vi "Magnetic Sweep 1.1.vi"() -> ()   [LabVIEW 2011]
panel:
  out "Intensity Graph 2":dbl[][](graph)
  in  "stop":bool
  out "error out 3":errorcluster
  out "error out 2":errorcluster
  out "Intensity Graph":dbl[][](graph)
  in  "Contour plot (ramp down)":path
  in  "Raw data (ramp down)":path
  out "Elapsed Time (s)":dbl
  out "Numeric":i32
  in  "error out":errorcluster
  out "Initial Temperature":string
  out "Zero field reached":bool
  out "Target field reached":bool
  in  "Upper limite":dbl
  in  "Temperature\nramping step":dbl
  in  "Heater range":i16(ring) items=["High", "Medium", "Low"]
  in  "D gain":dbl
  in  "I gain":dbl
  in  "P gain":dbl
  in  "Contour plot (ramp up)":path
  out "Time elapsed":string
  in  "Timer":bool caption="Reset"
  in  "date format":enum16{"short", "long", "abbreviated"}(ring)
  in  "Save":bool
  in  "Raw data (ramp  up)":path
  out "Temperature vs Time":cluster{dbl[], dbl[]}(graph)
  out "current time":timestamp
  out "Magnetic\nField":cluster{dbl[], dbl[]}(graph)
  out "Current Resistance":string
  out "Current Temperature":string
  out "Current Field":string
  out "Status":string
  in  "Field Sweep":bool
  in  "Start":bool
  out "Parameter\nSetup":string
  in  "Ramp rate":dbl
  in  "Traget Field":dbl
  out "Init Response":string
  in  "error in (no error)":errorcluster
  in  "IP Address":string
  in  "Ramp":bool
  in  "Update":bool
  in  "Ramp to Zero":bool
  in  "P Switch":bool
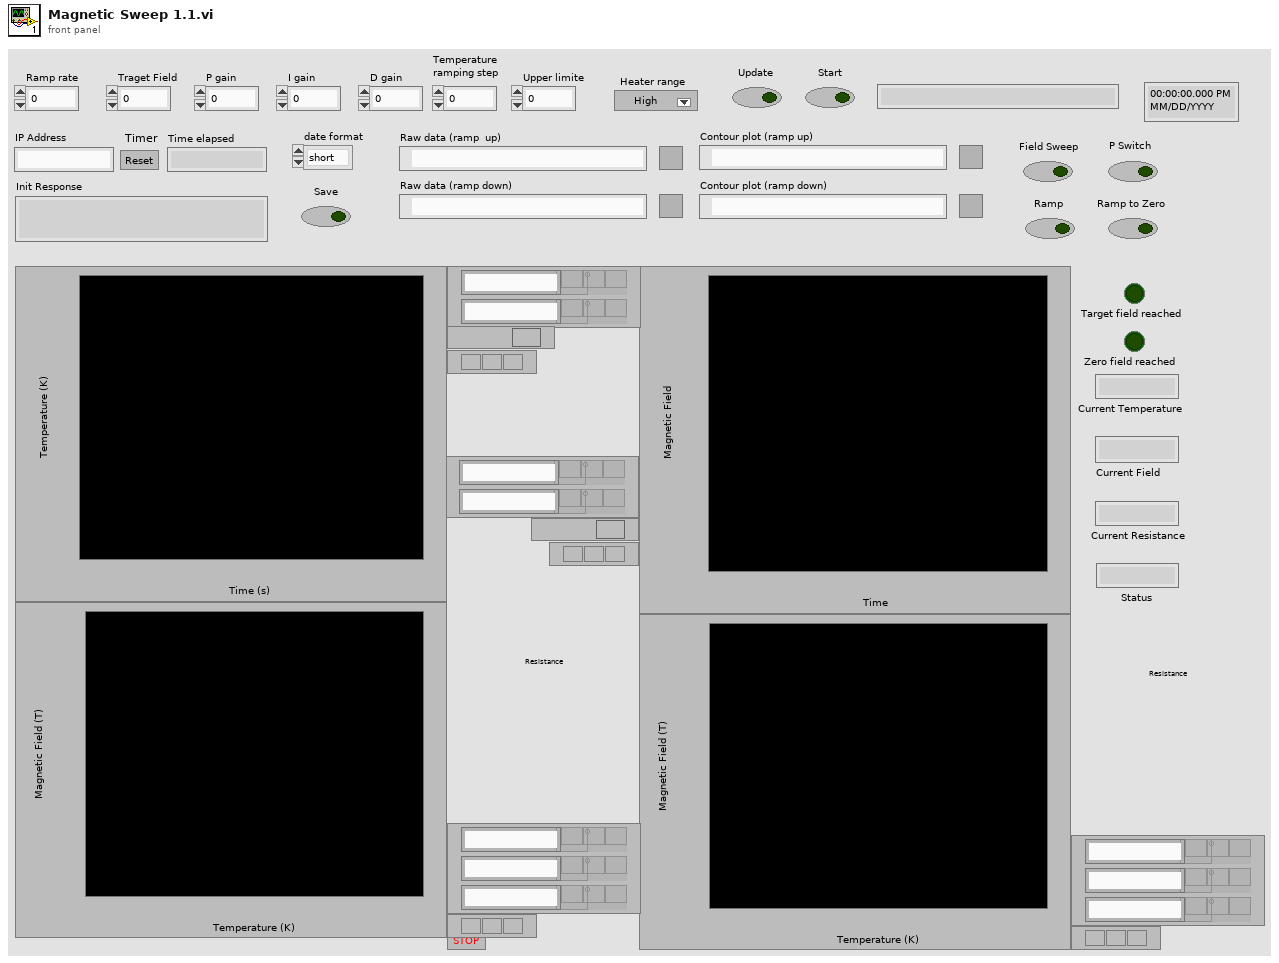
[diagram p1: front panel]
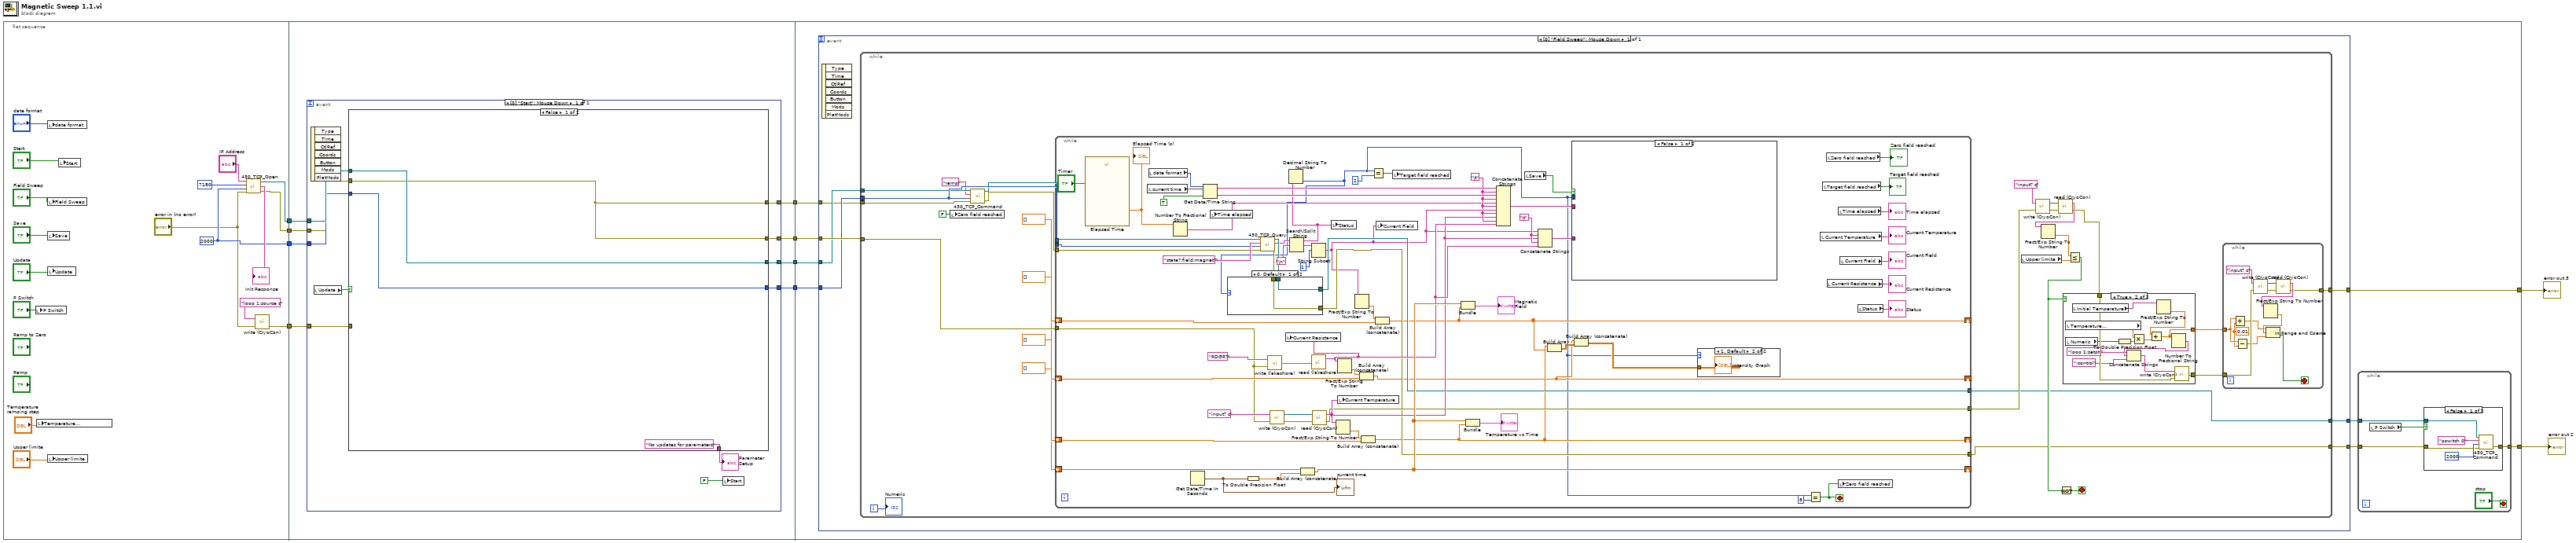
[diagram p0: block diagram]
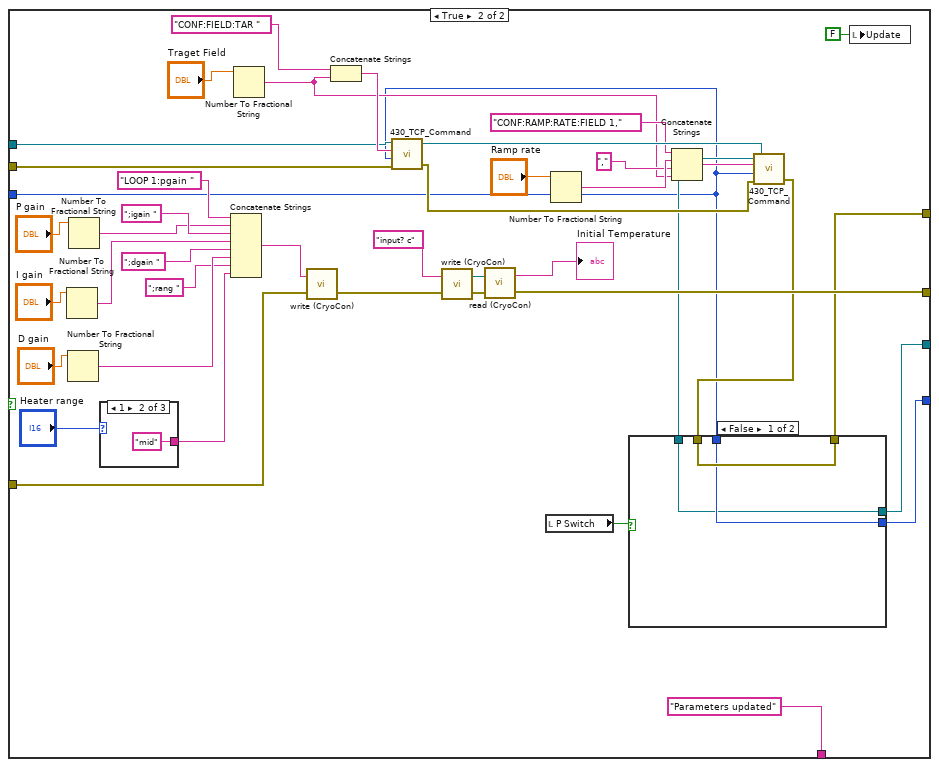
[diagram p2: hidden frame]
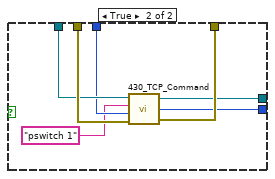
[diagram p3: hidden frame]
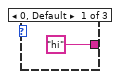
[diagram p4: hidden frame]
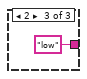
[diagram p5: hidden frame]
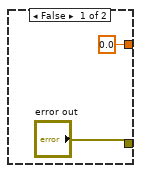
[diagram p7: hidden frame]
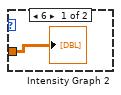
[diagram p8: hidden frame]
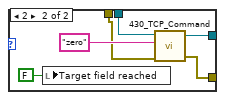
[diagram p9: hidden frame]
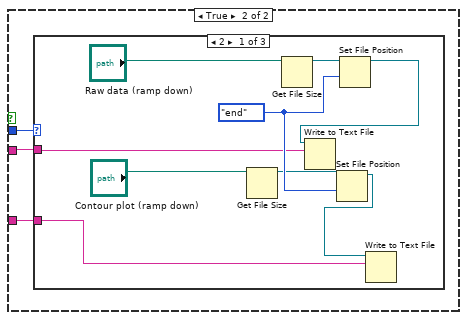
[diagram p10: hidden frame]
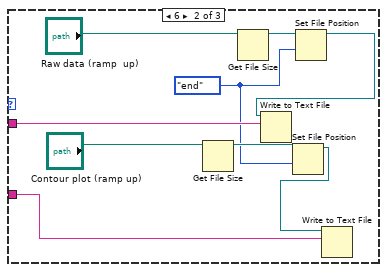
[diagram p11: hidden frame]
diagram:
  n1 = flat-sequence {
    tunnel: [w23] -> w10
    tunnel: [w22] -> w9
    tunnel: [w21] -> w8
    tunnel: [w17] -> w5
    tunnel: w10 -> [w35]
    tunnel: w9 -> [w34]
    tunnel: w8 -> [w33]
    tunnel: [w32] -> w7
    tunnel: [w31] -> w6
    tunnel: w5 -> [w30]
    tunnel: [w29] -> w4
    tunnel: [w28] -> w3
    tunnel: w7 -> [w113]
    tunnel: w6 -> [w112]
    tunnel: w4 -> [w111]
    tunnel: w3 -> [w110]
    tunnel: [w109] -> w2
    tunnel: [w107] -> w1
    frame #0 {
      w22 = 2000 ("Timeout")
      n2 = local write "P Switch"("P Switch") -> ()
      n3 = local write "Temperature\nramping step"("Temperature\nramping step") -> ()
      n4 = local write "date format"("date format") -> ()
      n5 = local write "Field Sweep"("Field Sweep") -> ()
      n6 = local write "Save"("Save") -> ()
      n7 = local write "Update"("Update") -> ()
      n8 = local write "Upper limite"("Upper limite") -> ()
      n9 = local write "Start"("Start") -> ()
      n10 = call "430_TCP_Open.vi"("IP Address"="IP Address", "TCP Port"=7180, "timeout ms (2000)"=w22, "error in (no error)"="error in (no error)") -> ("connection ID"=w23:refnum<k5>, "Init Response"=→"Init Response":string, "error out"=w21:errorcluster)  [unwired: 2 in]
      n11 = call "write (CryoCon).vi"("error in (no error)"="error in (no error)", "write buffer"="loop 1:source c") -> ("error out"=w17:errorcluster)  [unwired: 1 out]
    }
    frame #1 {
      n12 = event shown="[0] \"Start\": Mouse Down" {
        selector: _ -> [_]
        dyn-events: _ -> [_]
        timeout: _ -> [_]
        tunnel: w35 -> [w45]
        tunnel: w34 -> [w44]
        tunnel: w33 -> [w43]
        tunnel: [w42] -> w32
        tunnel: [w41] -> w31
        tunnel: w30 -> [w38]
        tunnel: [w37] -> w29
        tunnel: [w36] -> w28
        event "Start": Mouse Down {
          n13 = event-data() -> ()  [unwired: 1 in, 7 out]
          n14 = local read "Update"() -> (w46:bool)
          n15 = case shown="False" w46 {
            tunnel: w45 -> [w50 w90]
            tunnel: w44 -> [w49 w53]
            tunnel: w43 -> [w47 w78]
            tunnel: [w50 w52] -> w42
            tunnel: [w49 w51] -> w41
            tunnel: ["No updates for parameters" ("String") "Parameters updated" ("String")] -> w39
            tunnel: w38 -> [_ w67]
            tunnel: [w47 w59] -> w37
            tunnel: [w47 w55] -> w36
            frame False {
            }
            frame True {
              n16 = Number To Fractional String(number="I gain") -> (F-format string=w71:string)  [unwired: 3 in]
              n17 = Number To Fractional String(number="D gain") -> (F-format string=w69:string)  [unwired: 3 in]
              n18 = Number To Fractional String(number="P gain") -> (F-format string=w72:string)  [unwired: 3 in]
              n19 = case shown="1" "Heater range" {
                tunnel: ["hi" "mid" "low"] -> w64
                frame 0, Default {
                }
                frame 1 {
                }
                frame 2 {
                }
              }
              n20 = Concatenate Strings("LOOP 1:pgain " ("write buffer"), w72, ";igain " ("string"), w71, ";dgain " ("string"), w69, ";rang " ("string"), w64) -> (w68:string)
              n21 = Number To Fractional String(number="Traget Field") -> (F-format string=w79:string)  [unwired: 3 in]
              n22 = call "write (CryoCon).vi"("error in (no error)"=w67, "write buffer"=w68) -> ("error out"=w60:errorcluster)  [unwired: 1 out]
              n23 = Concatenate Strings("CONF:FIELD:TAR ", w79) -> (w91:string)
              n24 = call "430_TCP_Command.vi"("error in (no error)"=w78, "Timeout"=w53, "Command"=w91, "connection ID"=w90) -> ("error out"=w89:errorcluster, "connection ID out"=w85:refnum<k5>)  [unwired: 1 out]
              n25 = call "write (CryoCon).vi"("error in (no error)"=w60, "write buffer"="input? c") -> ("error out"=w63:errorcluster, "VISA resource name out"=w62:refnum<visa-resource-name>)
              n26 = call "read (CryoCon).vi"("error in (no error)"=w63, "VISA resource name"=w62) -> ("error out"=w59:errorcluster, "read buffer"=→"Initial Temperature":string)
              n27 = local read "P Switch"() -> (w57:bool)
              n28 = Number To Fractional String(number="Ramp rate") -> (F-format string=w83:string)  [unwired: 3 in]
              n29 = Concatenate Strings("CONF:RAMP:RATE:FIELD 1," ("string"), w83, "," ("string"), w79) -> (w86:string)
              n30 = call "430_TCP_Command.vi"("error in (no error)"=w89, "Timeout"=w53, "Command"=w86, "connection ID"=w85) -> ("error out"=w56:errorcluster, "connection ID out"=w54:refnum<k5>)  [unwired: 1 out]
              n31 = case shown="False" w57 {
                tunnel: w56 -> [w95 w102]
                tunnel: [w95 w101] -> w55
                tunnel: w54 -> [w93 w100]
                tunnel: w53 -> [w94 w99]
                tunnel: [w93 w98] -> w52
                tunnel: [w94 w97] -> w51
                frame False {
                }
                frame True {
                  n32 = call "430_TCP_Command.vi"("error in (no error)"=w102, "Timeout"=w99, "Command"="pswitch 1", "connection ID"=w100) -> ("error out"=w101:errorcluster, "bytes written"=w97:i32, "connection ID out"=w98:refnum<k5>)
                }
              }
              n33 = local write "Update"(FALSE ("Update")) -> ()
            }
          }
          "Parameter\nSetup" <- w39
          n34 = local write "Start"(FALSE ("Set Parameter")) -> ()
        }
      }
    }
    frame #2 {
      n35 = event shown="[0] \"Field Sweep\": Mouse Down" {
        selector: _ -> [_]
        dyn-events: _ -> [_]
        timeout: _ -> [_]
        tunnel: w113 -> [w130]
        tunnel: w112 -> [w129]
        tunnel: w111 -> [w131]
        tunnel: w110 -> [w128]
        tunnel: [w127] -> w109
        tunnel: [w126] -> w108
        tunnel: [w125] -> w106
        event "Field Sweep": Mouse Down {
          n36 = event-data() -> ()  [unwired: 1 in, 7 out]
          n37 = while {
            tunnel: w131 -> [w154]
            tunnel: w129 -> [w158]
            tunnel: w130 -> [w157]
            tunnel: w128 -> [w155]
            tunnel: [w134] -> w127
            tunnel: [w133] -> w126
            tunnel: [w132] -> w125
            i -> [w151]
            stop <- w136 stop-if-true
            n38 = local write "Zero field reached"(FALSE ("Zero field reached")) -> ()
            n39 = call "430_TCP_Command.vi"("error in (no error)"=w155, "Timeout"=w158, "Command"="ramp", "connection ID"=w157) -> ("error out"=w159:errorcluster, "connection ID out"=w156:refnum<k5>)  [unwired: 1 out]
            n40 = while {
              shift-right: [w190] -> _
              shift-left: dbl[] [] -> [w242]
              shift-right: [w191] -> _
              shift-left: dbl[] [] -> [w247]
              shift-right: [w188] -> _
              shift-left: dbl[] [] -> [w244]
              shift-right: [w237] -> _
              shift-left: dbl[] [] -> [w238]
              tunnel: w159 -> [w226]
              tunnel: w158 -> [w202]
              tunnel: w156 -> [w225]
              tunnel: w154 -> [w219]
              tunnel: [w212] -> w137
              tunnel: [w200] -> w133
              tunnel: [w199] -> w132
              stop <- w204 stop-if-true
              w230 = "\t"
              w231 = "\t"
              n41 = call "Elapsed Time"("Reset"="Timer") -> ("Elapsed Time (s)"=w217:dbl)  [unwired: 11 in, 7 out]
              "Elapsed Time (s)" <- w217
              n42 = local read "current time"() -> (w228:timestamp)
              n43 = local read "date format"() -> (w220:enum16{"short", "long", "abbreviated"})
              n44 = Number To Fractional String(number=w217) -> (F-format string=w223:string)  [unwired: 3 in]
              n45 = Get Date/Time In Seconds() -> (seconds since 1Jan1904=w216:timestamp)
              "current time" <- w216
              n46 = Get Date/Time String(date format (0)=w220, seconds (now)=w228, want seconds? (F)=TRUE) -> (date string=w233:string, time string=w232:string)
              n47 = local write "Time elapsed"(w223) -> ()
              n48 = To Double Precision Float(number=w216) -> (double precision float=w239:dbl)
              n49 = call "430_TCP_Query.vi"("error in (no error)"=w226, "Timeout"=w202, "Command"="state?;field:magnet?", "connection ID"=w225) -> ("error out"=w214:errorcluster, "Response"=w198:string, "connection ID out"=w203:refnum<k5>)  [unwired: 3 in, 2 out]
              n50 = call "write (lakeshore).vi"("error in (no error)"=w219, "write buffer"="RDGR?") -> ("error out"=w246:errorcluster)
              n51 = call "write (CryoCon).vi"("error in (no error)"=w219, "write buffer"="input? c") -> ("error out"=w248:errorcluster, "VISA resource name out"=w249:refnum<visa-resource-name>)
              n52 = Search/Split String(string=w198, search string/char (-)="\n") -> (substring before match=w197:string, match + rest of string=w196:string)  [unwired: 1 in, 1 out]
              n53 = Decimal String To Number(string=w197) -> (number=w187:i32)  [unwired: 2 in, 1 out]
              n54 = case shown="0, Default" w187 {
                tunnel: w214 -> [w255 w260]
                tunnel: [w255 w259] -> w199
                tunnel: w203 -> [w254 w257]
                tunnel: [w254 w256] -> w200
                frame 0, Default {
                }
                frame 2 {
                  n55 = local write "Target field reached"(FALSE ("Target field reached")) -> ()
                  n56 = call "430_TCP_Command.vi"("error in (no error)"=w260, "Command"="zero", "connection ID"=w257) -> ("error out"=w259:errorcluster, "connection ID out"=w256:refnum<k5>)  [unwired: 1 in, 1 out]
                }
              }
              n57 = Build Array (concatenate)(w238, w239) -> (w237:dbl[])
              n58 = call "read (lakeshore).vi"("error in (no error)"=w246) -> ("read buffer"=w222:string)  [unwired: 1 out]
              n59 = local write "Current Resistance"(w222) -> ()
              n60 = String Subset(string=w196, offset (0)=1) -> (substring=w194:string)  [unwired: 1 in]
              n61 = call "read (CryoCon).vi"("error in (no error)"=w248, "VISA resource name"=w249) -> ("error out"=w212:errorcluster, "read buffer"=w221:string)
              n62 = local write "Status"(w197) -> ()
              n63 = Fract/Exp String To Number(string=w221) -> (number=w241:dbl)  [unwired: 3 in, 1 out]
              n64 = Fract/Exp String To Number(string=w222) -> (number=w240:dbl)  [unwired: 3 in, 1 out]
              n65 = local write "Current Temperature"(w221) -> ()
              n66 = Fract/Exp String To Number(string=w194) -> (number=w243:dbl)  [unwired: 3 in, 1 out]
              n67 = Build Array (concatenate)(w240, w244) -> (w188:dbl[])
              n68 = Build Array (concatenate)(w241, w247) -> (w191:dbl[])
              n69 = Equal?(x=w187, y=2) -> (x = y?=w224:bool)
              n70 = Build Array (concatenate)(w243, w242) -> (w190:dbl[])
              n71 = local write "Current Field"(w194) -> ()
              n72 = local write "Target field reached"(w224) -> ()
              n73 = Bundle(w237, w190) -> (→"Magnetic\nField":cluster{dbl[], dbl[]})  [unwired: 1 in]
              n74 = Bundle(w237, w191) -> (→"Temperature vs Time":cluster{dbl[], dbl[]})  [unwired: 1 in]
              n75 = Concatenate Strings(w233, w231, w232, w231, w223, w231, w194, w231, w221, w231, w222) -> (w236:string)
              n76 = local read "Save"() -> (w215:bool)
              n77 = Concatenate Strings(w194, w230, w221, w230, w222) -> (w229:string)
              n78 = Build Array(w191, w190) -> (w201:dbl[][])
              n79 = case shown="False" w215 {
                tunnel: w236 -> [_ w264]
                tunnel: w229 -> [_ w263]
                tunnel: w187 -> [_ w262]
                frame False {
                }
                frame True {
                  n80 = case shown="2" w262 {
                    tunnel: w264 -> [w266 w282 _]
                    tunnel: w263 -> [w265 w276 _]
                    frame 2 {
                      w272 = enum16{"start", "end", "current"}."end" ("from (0:start)")
                      n81 = Get File Size(file="Contour plot (ramp down)") -> (refnum out=w271:refnum<file>)  [unwired: 1 in, 2 out]
                      n82 = Get File Size(file="Raw data (ramp down)") -> (refnum out=w268:refnum<file>)  [unwired: 1 in, 2 out]
                      n83 = Set File Position(refnum=w271, from (0:start)=w272) -> (refnum out=w273:refnum<file>)  [unwired: 2 in, 1 out]
                      n84 = Set File Position(refnum=w268, from (0:start)=w272) -> (refnum out=w269:refnum<file>)  [unwired: 2 in, 1 out]
                      n85 = Write to Text File(file (use dialog)=w269, text=w266) -> ()  [unwired: 2 in, 3 out]
                      n86 = Write to Text File(file (use dialog)=w273, text=w265) -> ()  [unwired: 2 in, 3 out]
                    }
                    frame 6 {
                      w275 = enum16{"start", "end", "current"}."end" ("from (0:start)")
                      n87 = Get File Size(file="Contour plot (ramp up)") -> (refnum out=w277:refnum<file>)  [unwired: 1 in, 2 out]
                      n88 = Get File Size(file="Raw data (ramp  up)") -> (refnum out=w280:refnum<file>)  [unwired: 1 in, 2 out]
                      n89 = Set File Position(refnum=w277, from (0:start)=w275) -> (refnum out=w274:refnum<file>)  [unwired: 2 in, 1 out]
                      n90 = Set File Position(refnum=w280, from (0:start)=w275) -> (refnum out=w279:refnum<file>)  [unwired: 2 in, 1 out]
                      n91 = Write to Text File(file (use dialog)=w279, text=w282) -> ()  [unwired: 2 in, 3 out]
                      n92 = Write to Text File(file (use dialog)=w274, text=w276) -> ()  [unwired: 2 in, 3 out]
                    }
                    frame Default {
                    }
                  }
                }
              }
              n93 = Build Array (concatenate)(w188, w201) -> (w189:dbl[][])
              n94 = case shown="1, Default" w187 {
                tunnel: w189 -> [w252 w253]
                frame 6 {
                  "Intensity Graph 2" <- w252
                }
                frame 1, Default {
                  "Intensity Graph" <- w253
                }
              }
              n95 = Equal?(x=w187, y=8) -> (x = y?=w204:bool)
              n96 = local read "Current Temperature"() -> (→"Current Temperature":string)
              n97 = local read "Target field reached"() -> (→"Target field reached":bool)
              n98 = local read "Zero field reached"() -> (→"Zero field reached":bool)
              n99 = local read "Current Resistance"() -> (→"Current Resistance":string)
              n100 = local read "Time elapsed"() -> (→"Time elapsed":string)
              n101 = local write "Zero field reached"(w204) -> ()
              n102 = local read "Current Field"() -> (→"Current Field":string)
              n103 = local read "Status"() -> (→"Status":string)
            }
            n104 = local read "Upper limite"() -> (w139:dbl)
            n105 = call "write (CryoCon).vi"("error in (no error)"=w137, "write buffer"="input? c") -> ("error out"=w142:errorcluster, "VISA resource name out"=w143:refnum<visa-resource-name>)
            n106 = call "read (CryoCon).vi"("error in (no error)"=w142, "VISA resource name"=w143) -> ("error out"=w140:errorcluster, "read buffer"=w141:string)
            n107 = Fract/Exp String To Number(string=w141) -> (number=w138:dbl)  [unwired: 3 in, 1 out]
            n108 = Less Or Equal?(x=w138, y=w139) -> (x <= y?=w135:bool)
            n109 = Not(x=w135) -> (.not. x?=w136:bool)
            n110 = case shown="True" w135 {
              tunnel: w140 -> [_ w183]
              tunnel: ["error out" w180] -> w153
              tunnel: [0.0 w179] -> w152
              frame False {
              }
              frame True {
                n111 = local read "Temperature\nramping step"() -> (w177:dbl)
                n112 = local read "Numeric"() -> (w175:i32)
                n113 = local read "Initial Temperature"() -> (w182:string)
                n114 = To Double Precision Float(number=w175) -> (double precision float=w176:dbl)
                n115 = Multiply(x=w177, y=w176) -> (x*y=w178:dbl)
                n116 = Fract/Exp String To Number(string=w182) -> (number=w181:dbl)  [unwired: 3 in, 1 out]
                n117 = Add(x=w181, y=w178) -> (x+y=w179:dbl)
                n118 = Number To Fractional String(number=w179) -> (F-format string=w184:string)  [unwired: 3 in]
                n119 = Concatenate Strings("loop 1:setpt " ("write buffer"), w184, ";control" ("string")) -> (w186:string)
                n120 = call "write (CryoCon).vi"("error in (no error)"=w183, "write buffer"=w186) -> ("error out"=w180:errorcluster)  [unwired: 1 out]
              }
            }
            n121 = while {
              tunnel: w153 -> [w170]
              tunnel: w152 -> [w165]
              tunnel: [w160] -> w134
              stop <- w161 stop-if-true
              w162 = 0.01 ("y")
              n122 = Add(x=w165, y=w162) -> (x+y=w164:dbl)
              n123 = Subtract(x=w165, y=w162) -> (x-y=w163:dbl)
              n124 = call "write (CryoCon).vi"("error in (no error)"=w170, "write buffer"="input? c") -> ("error out"=w169:errorcluster, "VISA resource name out"=w171:refnum<visa-resource-name>)
              n125 = call "read (CryoCon).vi"("error in (no error)"=w169, "VISA resource name"=w171) -> ("error out"=w160:errorcluster, "read buffer"=w167:string)
              n126 = Fract/Exp String To Number(string=w167) -> (number=w166:dbl)  [unwired: 3 in, 1 out]
              n127 = In Range and Coerce(upper limit=w164, x=w166, lower limit=w163) -> (In Range?=w161:bool)  [unwired: 1 out]
            }
            "Numeric" <- w151
          }
        }
      }
      n128 = while {
        tunnel: w108 -> [w118]
        tunnel: [w116] -> w107
        tunnel: w106 -> [w115]
        stop <- "stop" stop-if-true
        n129 = local read "P Switch"() -> (w117:bool)
        n130 = case shown="False" w117 {
          tunnel: w118 -> [w122 _]
          tunnel: [w120 w124] -> w116
          tunnel: w115 -> [w119 w124]
          frame False {
            n131 = call "430_TCP_Command.vi"("error in (no error)"=w119, "Timeout"=2000, "Command"="pswitch 0", "connection ID"=w122) -> ("error out"=w120:errorcluster)  [unwired: 2 out]
          }
          frame True {
          }
        }
      }
    }
  }
  "error out 2" <- w1
  "error out 3" <- w2
